vi "x.vi"() -> ()   [LabVIEW 2018]
uses:
  <vilib>/myRIO/Instrument Drivers/Onboard IO/I2C/typedefs/I2C User Configuration.ctl
  <vilib>/myRIO/Instrument Drivers/Onboard IO/I2C/typedefs/I2C Transfer Rate.ctl
  <vilib>/myRIO/Instrument Drivers/Onboard IO/I2C/typedefs/I2C Reference.ctl
  <vilib>/myRIO/Common/Instrument Driver Framework/Utilities/typedefs/myRIO Generic Hardware Reference.ctl
  <vilib>/myRIO/Common/Instrument Driver Framework/Utilities/typedefs/Hardware Version Enum.ctl
  <vilib>/myRIO/Common/Instrument Driver Framework/Utilities/typedefs/myRIO v1.0 Reference.ctl
  <vilib>/myRIO/Common/Instrument Driver Framework/Utilities/typedefs/Generic FPGA Reference.ctl
  <vilib>/myRIO/Common/Instrument Driver Framework/myRIO v1.0/I2C/typedefs/I2C Channels Enum.ctl
  <vilib>/myRIO/Instrument Drivers/Onboard IO/I2C/typedefs/I2C Configuration.ctl
  <vilib>/userdefined/High Color/nirio_resource_hc.ctl
  <vilib>/myRIO/Common/Instrument Driver Framework/Utilities/vis/Is FPGA Ref Available.vi
  <vilib>/myRIO/Common/Instrument Driver Framework/myRIO v1.0/I2C/vis/myRIO v1.1 Open I2C.vi
  <vilib>/myRIO/Instrument Drivers/Onboard IO/I2C/vis/Configure.vi
  <vilib>/myRIO/Instrument Drivers/Onboard IO/I2C/vis/Write Read.vi
  <vilib>/myRIO/Instrument Drivers/Onboard IO/I2C/vis/Write.vi
  <vilib>/myRIO/Common/Instrument Driver Framework/Utilities/vis/Validate Channels.vi
  <vilib>/myRIO/Common/Instrument Driver Framework/myRIO v1.0/I2C/vis/myRIO v1.0 Reserve I2C.vi
  <vilib>/myRIO/Common/Instrument Driver Framework/myRIO v1.0/I2C/vis/myRIO v1.0 Build MUX Configuration I2C.vi
  <vilib>/myRIO/Common/Instrument Driver Framework/myRIO v1.0/Resource Manager/vis/myRIO v1.0 Reserve Channel List.vi
  <vilib>/myRIO/Common/Instrument Driver Framework/myRIO v1.0/Resource Manager/vis/myRIO v1.0 Create Configuration List.vi
  <vilib>/myRIO/Common/Instrument Driver Framework/myRIO v1.0/Resource Manager/vis/myRIO v1.0 Reserve Channel.vi
  <vilib>/myRIO/Common/Instrument Driver Framework/myRIO v1.0/Resource Manager/vis/myRIO v1.0 Unreserve Channel.vi
  <vilib>/myRIO/Common/Instrument Driver Framework/myRIO v1.0/Resource Manager/vis/myRIO v1.0 Build Mutex Name.vi
  <vilib>/Utility/VariantDataType/GetNumericInfo.vi
  <vilib>/Utility/error.llb/Error Cluster From Error Code.vi
  <vilib>/myRIO/Common/Instrument Driver Framework/myRIO v1.0/myRIO v1.1 Open.vi
  <vilib>/myRIO/Common/Instrument Driver Framework/Utilities/vis/IO Manager.vi
  <vilib>/myRIO/Common/Instrument Driver Framework/Utilities/vis/Configuration Manager.vi
  <vilib>/myRIO/Common/Instrument Driver Framework/myRIO v1.0/Resource Manager/vis/myRIO v1.0 Configure IO.vi
  <vilib>/myRIO/Common/Instrument Driver Framework/myRIO v1.0/myRIO v1.0 Close.vi
  <vilib>/myRIO/Common/Instrument Driver Framework/myRIO v1.0/I2C/vis/myRIO v1.0 Configure I2C.vi
  <vilib>/myRIO/Common/Instrument Driver Framework/myRIO v1.0/I2C/vis/myRIO v1.0 Write I2C.vi
  <vilib>/myRIO/Common/Instrument Driver Framework/myRIO v1.0/I2C/vis/myRIO v1.0 Read I2C.vi
  <vilib>/myRIO/Express VI/Onboard IO/I2C/I2C Express VI.xnode
  <vilib>/myRIO/Instrument Drivers/Onboard IO/I2C/vis/myRIO I2C Open.xnode
  <vilib>/myRIO/Instrument Drivers/Onboard IO/I2C/I2C.lvlib
panel:
  out "register":u8 format="%02x"
  in  "Register":T1(ring)
  in  "Gain":enum8{"1x", "4x", "16x", "60x"}(ring)
  out "Data":u16
  out "Bytes Read":u8[](array[numeric])
  out "Not connected":bool
  in  "Stop Button":bool
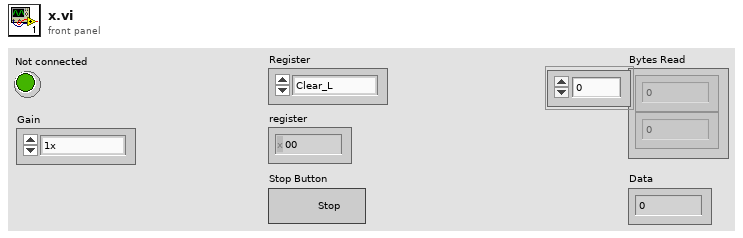
[diagram p1: front panel]
types:
  T1 = enum8{"Clear_L", "Clear_H", "Red_L", "Red_H", "Green_L", "Green_H", "Blue_L", "Blue_H"}
  T2 = typedef "I2C.lvlib/I2C Reference.ctl" = cluster{"myRIO Reference":T3, "I2C Channels Enum":T7, "I2C Configuration":T8}
  T3 = typedef "myRIO Generic Hardware Reference.ctl" = cluster{"myRIO Model":T4, "myRIO Hardware Reference":T5}
  T4 = typedef "Hardware Version Enum.ctl" = enum16{"Unknown", "myRIO-1900", "myRIO-1950", "roboRIO", "NI ELVIS RIO CM", "ELVIS III"}
  T5 = typedef "myRIO v1.0 Reference.ctl" = cluster{"Generic FPGA Reference":T6, "Allow multiple opens":bool}
  T6 = typedef "Generic FPGA Reference.ctl" = refnum<k20>
  T7 = typedef "I2C Channels Enum.ctl" = enum16{"Not Connected", "A/I2C", "B/I2C", "I2C/I2C"}
  T8 = typedef "I2C.lvlib/I2C Configuration.ctl" = cluster{"I2C Transfer Rate":T9}
  T9 = typedef "I2C.lvlib/I2C Transfer Rate.ctl" = enum16{"Standard mode (100 kbps)", "Fast mode (400 kbps)"}
  T10 = typedef "I2C.lvlib/I2C User Configuration.ctl" = cluster{"I2C Transfer Rate":T9}
  T11 = typedef "nirio_resource_hc.ctl" = tag
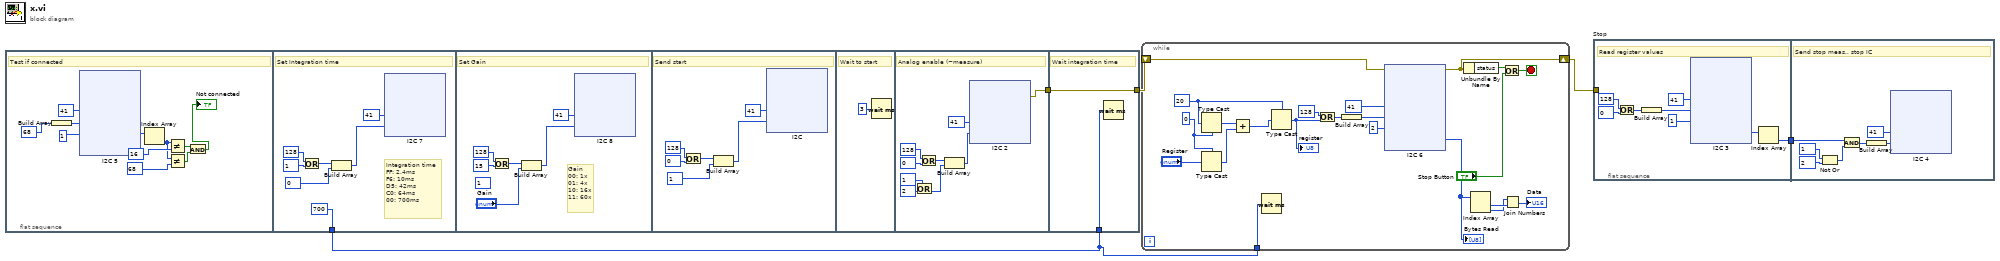
[diagram p0: block diagram]
diagram:
  n1 = flat-sequence {
    tunnel: [u32 700] -> w1
    tunnel: [w191] -> w4
    tunnel: [w239] -> w3
    tunnel: w4 -> [w239]
    tunnel: w1 -> [w238]
    frame #0 {
      # "Test if connected"
      n2 = Build Array(u8 68 ("Slave Address (7-bit)")) -> (w6:u8[])
      n3 = xnode "I2C 5"("Slave Address (7-bit)"=u8 41, "Bytes to Write"=w6, "Byte Count"=u32 1) -> ("Bytes Read"=w15:u8[])  [unwired: 1 in, 1 out]
      n4 = Index Array(array=w15) -> (element=w13:u8)  [unwired: 1 in]
      n5 = Not Equal?(x=w13, y=u8 16 ("Slave Address (7-bit)")) -> (x != y?=w11:bool)
      n6 = Not Equal?(x=w13, y=u8 68 ("Slave Address (7-bit)")) -> (x != y?=w10:bool)
      n7 = And(x=w11, y=w10) -> (x .and. y?=→"Not connected":bool)
    }
    frame #1 {
      # "Integration time\nFF: 2.4ms\nF6: 10ms\nD5: 42ms\nC0: 64ms\n00: 700ms"
      # "Set Integration time"
      n8 = Or(x=u8 128 ("Slave Address (7-bit)"), y=u8 1 ("Slave Address (7-bit)")) -> (x .or. y?=w61:u8)
      n9 = Build Array(w61, u8 0 ("Slave Address (7-bit)")) -> (w62:u8[])
      n10 = xnode "I2C 7"("Slave Address (7-bit)"=u8 41, "Bytes to Write"=w62) -> ()  [unwired: 1 in, 1 out]
    }
    frame #2 {
      (unwired) u8 1 ("Slave Address (7-bit)")
      # "Gain\n00: 1x\n01: 4x\n10: 16x\n11: 60x"
      # "Set Gain"
      n11 = Or(x=u8 128 ("Slave Address (7-bit)"), y=u8 15 ("Slave Address (7-bit)")) -> (x .or. y?=w104:u8)
      n12 = Build Array(w104, "Gain") -> (w103:u8[])
      n13 = xnode "I2C 8"("Slave Address (7-bit)"=u8 41, "Bytes to Write"=w103) -> ()  [unwired: 1 in, 1 out]
    }
    frame #3 {
      # "Send start"
      n14 = Or(x=u8 128 ("Slave Address (7-bit)"), y=u8 0 ("Slave Address (7-bit)")) -> (x .or. y?=w148:u8)
      n15 = Build Array(w148, u8 1 ("Slave Address (7-bit)")) -> (w147:u8[])
      n16 = xnode "I2C"("Slave Address (7-bit)"=u8 41, "Bytes to Write"=w147) -> ()  [unwired: 1 in, 1 out]
    }
    frame #4 {
      # "Wait to start"
      n17 = Wait (ms)(milliseconds to wait=u32 3) -> ()  [unwired: 1 out]
    }
    frame #5 {
      # "Analog enable (~measure)"
      n18 = Or(x=u8 1 ("Slave Address (7-bit)"), y=u8 2 ("Slave Address (7-bit)")) -> (x .or. y?=w193:u8)
      n19 = Or(x=u8 128 ("Slave Address (7-bit)"), y=u8 0 ("Slave Address (7-bit)")) -> (x .or. y?=w198:u8)
      n20 = Build Array(w198, w193) -> (w194:u8[])
      n21 = xnode "I2C 2"("Slave Address (7-bit)"=u8 41, "Bytes to Write"=w194) -> ("error out"=w191:errorcluster)  [unwired: 1 in]
    }
    frame #6 {
      # "Wait integration time"
      n22 = Wait (ms)(milliseconds to wait=w238) -> ()  [unwired: 1 out]
    }
  }
  n23 = while {
    shift-right: [w254] -> w2
    shift-left: w3 -> [w255]
    tunnel: w1 -> [w240]
    stop <- w253 stop-if-true
    w242 = u16 0
    w243 = u8 20 ("Slave Address (7-bit)")
    n24 = Type Cast(type=w242, x=w243) -> (*(type *) &x=w241:u16)
    n25 = Type Cast(type=w242, x="Register") -> (*(type *) &x=w244:u16)
    n26 = Add(x=w241, y=w244) -> (x+y=w247:u16)
    n27 = Wait (ms)(milliseconds to wait=w240) -> ()  [unwired: 1 out]
    n28 = Type Cast(type=w243, x=w247) -> (*(type *) &x=w246:u8)
    "register" <- w246
    n29 = Or(x=u8 128 ("Slave Address (7-bit)"), y=w246) -> (x .or. y?=w258:u8)
    n30 = Build Array(w258) -> (w259:u8[])
    n31 = xnode "I2C 6"("Slave Address (7-bit)"=u8 41, "Bytes to Write"=w259, "Byte Count"=u32 2, "error in (no error)"=w255) -> ("Bytes Read"=w251:u8[], "error out"=w254:errorcluster)
    "Bytes Read" <- w251
    n32 = Unbundle By Name(w254) -> ("status"=w252:bool)
    n33 = Index Array(array=w251) -> (element #1=w250:u8, element #2=w249:u8)  [unwired: 2 in]
    n34 = Or(x=w252, y="Stop Button") -> (x .or. y?=w253:bool)
    n35 = Join Numbers(hi=w249, lo=w250) -> ((hi.lo)=→"Data":u16)
  }
  n36 = flat-sequence "Stop" {
    tunnel: [w302] -> w5
    tunnel: w2 -> [_]
    tunnel: w5 -> [w352]
    frame #0 {
      # "Read register values"
      n37 = Or(x=u8 128 ("Slave Address (7-bit)"), y=u8 0 ("Slave Address (7-bit)")) -> (x .or. y?=w307:u8)
      n38 = Build Array(w307) -> (w305:u8[])
      n39 = xnode "I2C 3"("Slave Address (7-bit)"=u8 41, "Bytes to Write"=w305, "Byte Count"=u32 1) -> ("Bytes Read"=w303:u8[])  [unwired: 1 in, 1 out]
      n40 = Index Array(array=w303) -> (element=w302:u8)  [unwired: 1 in]
    }
    frame #1 {
      # "Send stop meas., stop IC"
      n41 = Not Or(1:u8 2 ("Slave Address (7-bit)"), 2:u8 1 ("Slave Address (7-bit)")) -> (0:w353:u8)
      n42 = And(x=w352, y=w353) -> (x .and. y?=w351:u8)
      n43 = Build Array(w351) -> (w350:u8[])
      n44 = xnode "I2C 4"("Slave Address (7-bit)"=u8 41, "Bytes to Write"=w350) -> ()  [unwired: 1 in, 1 out]
    }
  }
